vi "Write Root UID.vi"(8 "error in (no error)":errorcluster, 10 "Root UID":string, 11 "Base Tree in":refnum<class "Base Tree.lvclass">) -> (0 "error out":errorcluster, 3 "Base Tree out":refnum<class "Base Tree.lvclass">)   [LabVIEW 2017, in "Browser Core.lvlib" / "Base Tree.lvclass"]
uses:
  Base Tree.lvclass
  Base Tree.lvclass/Base Tree.ctl
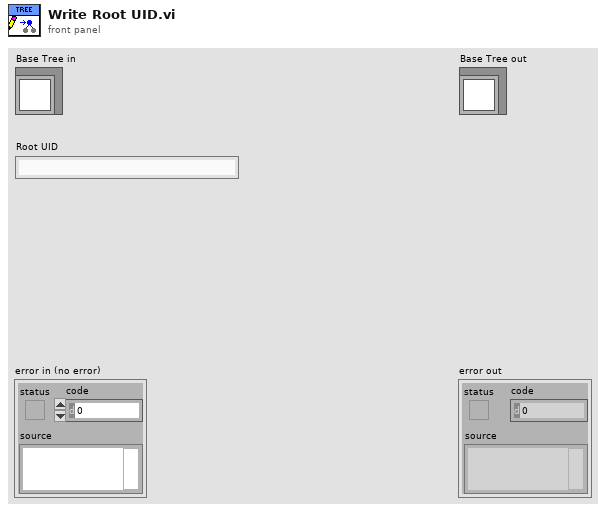
[diagram p1: front panel]
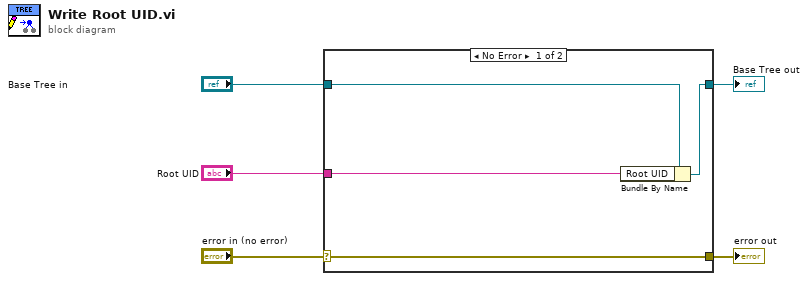
[diagram p0: block diagram]
diagram:
  n1 = case shown="No Error" "error in (no error)" {
    selector: "error in (no error)" -> [w9 w10]
    tunnel: [w9 w10] -> w4
    tunnel: [w7 w11] -> w2
    tunnel: "Base Tree in" -> [w8 w11]
    tunnel: "Root UID" -> [w6 _]
    frame No Error {
      n2 = Bundle By Name(cluster=w8, "Root UID"=w6) -> (w7:refnum<class "Base Tree.lvclass">)
    }
    frame Error {
    }
  }
  "error out" <- w4
  "Base Tree out" <- w2
